vi "get Data.vi"(11 "Memory in":refnum<class "Memory.lvclass">) -> (3 "Data":u8[](array[numeric]))   [LabVIEW 2021, in "Memory.lvclass"]
uses:
  Memory.lvclass
  Memory.lvclass/Memory.ctl
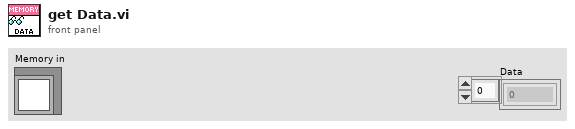
[diagram p1: front panel]
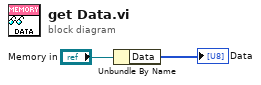
[diagram p0: block diagram]
diagram:
  n1 = Unbundle By Name("Memory in") -> ("Data"=→"Data":u8[])
